vi "Configure Auto Increment Start End Address.vi"(8 "error in (no error)":errorcluster, 9 "End Address (000)":i32 min=0 max=511 step=1 format="%03.0f", 10 "Start Address (000)":i32 min=0 max=511 step=1 format="%03.0f", 11 "VISA resource name":refnum<visa-resource-name>) -> (0 "error out":errorcluster, 3 "VISA resource name out":refnum<visa-resource-name>)   [LabVIEW 2018, in "EFD Ultimus V.lvlib"]
doc: "Downloads the auto increment start and end addresses.\n\nHost Format: SS--SsssEeee\n sss: Start Address 000 - 511 \n eee: End Address 000 - 511"
uses:
  EFD Ultimus V.lvlib
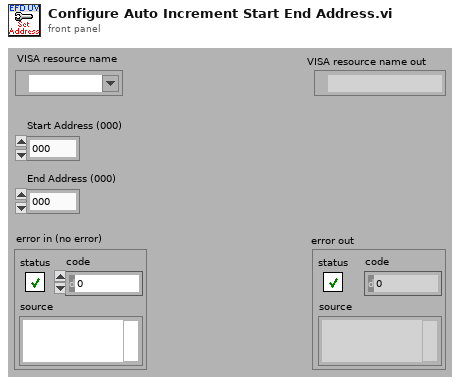
[diagram p1: front panel]
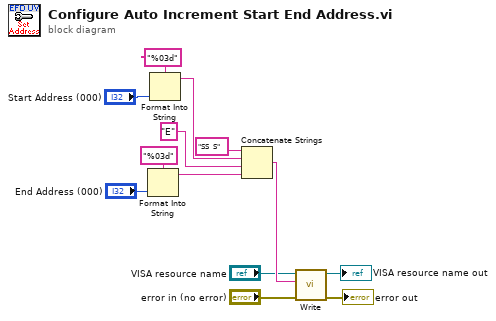
[diagram p0: block diagram]
diagram:
  n1 = Format Into String(format string="%03d", "End Address (000)") -> (resulting string=w3:string)  [unwired: 2 in, 1 out]
  n2 = Format Into String(format string="%03d", "Start Address (000)") -> (resulting string=w6:string)  [unwired: 2 in, 1 out]
  n3 = Concatenate Strings("SS  S" ("string"), w6, "E" ("string"), w3) -> (w11:string)
  n4 = call "Write.vi"("error in (no error)"="error in (no error)", "Command To Write"=w11, "VISA resource name"="VISA resource name") -> ("error out"=→"error out":errorcluster, "VISA resource name out"=→"VISA resource name out":refnum<visa-resource-name>)  [unwired: 7 out]
